vi "getShiftNdDate.vi"(8 "Error In":errorcluster) -> (0 "Error Out":errorcluster, 2 "Production Date":string, 3 "Shift":string)   [LabVIEW 2018]
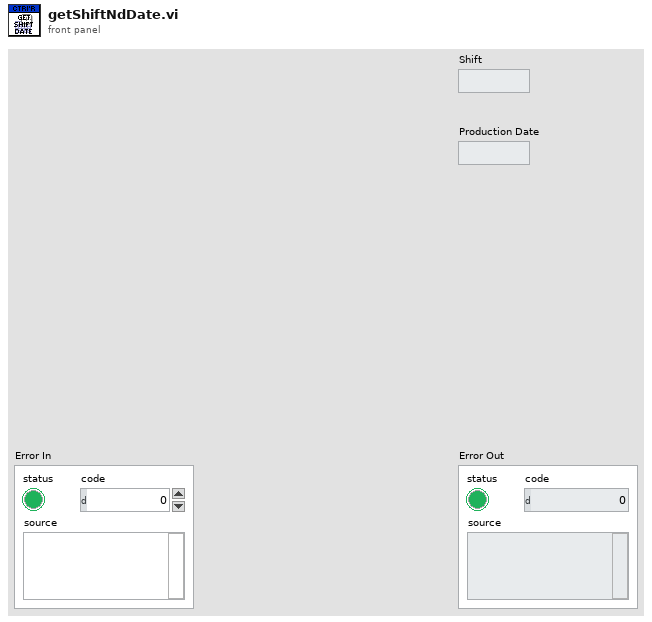
[diagram p1: front panel]
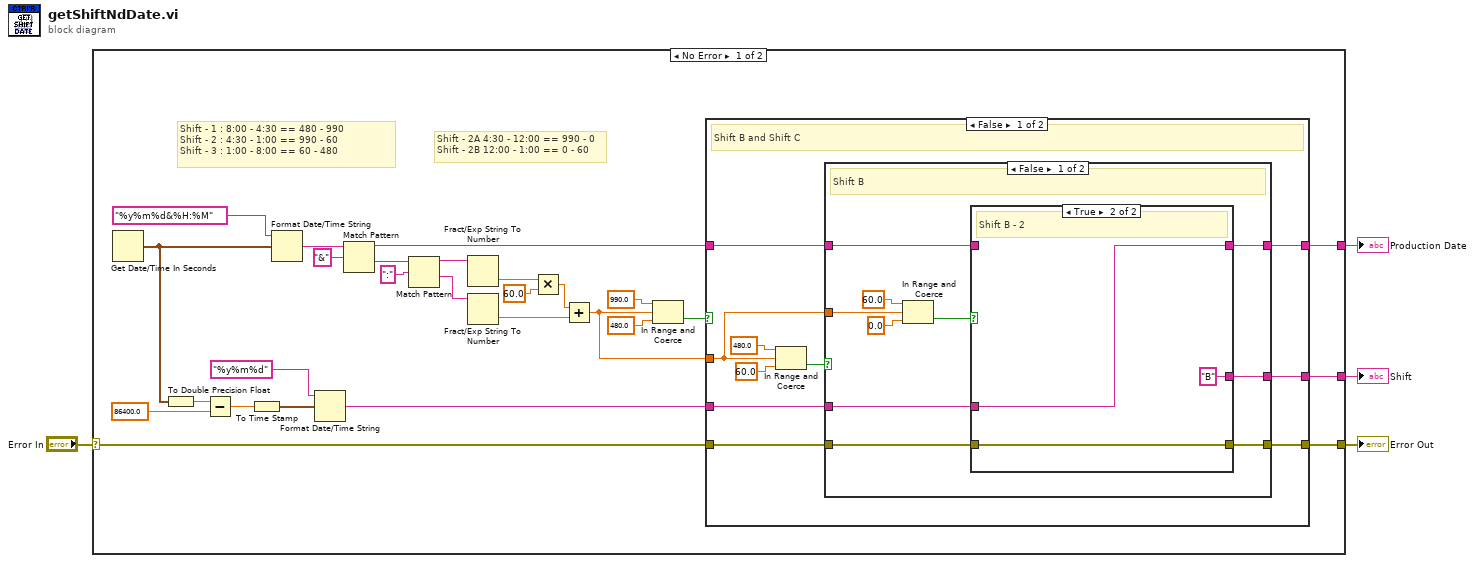
[diagram p0: block diagram]
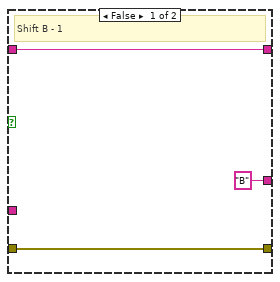
[diagram p2: hidden frame]
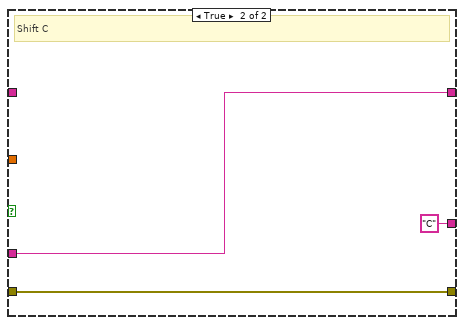
[diagram p3: hidden frame]
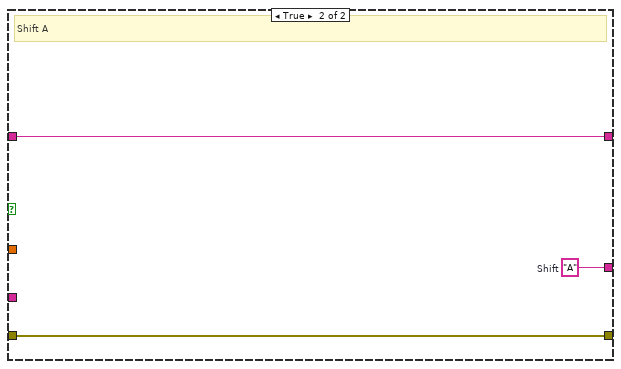
[diagram p4: hidden frame]
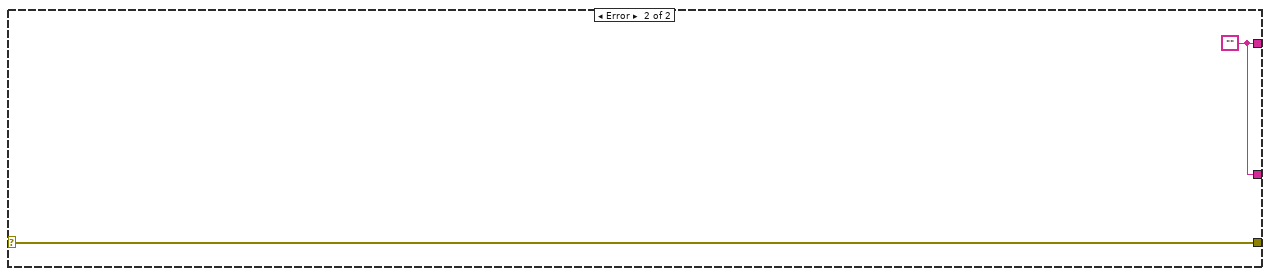
[diagram p5: hidden frame]
diagram:
  n1 = case shown="No Error" "Error In" {
    selector: "Error In" -> [w9 w65]
    tunnel: [w8 w65] -> w3
    tunnel: [w7 w64] -> w2
    tunnel: [w6 w64] -> w1
    frame No Error {
      # "Shift - 2A 4:30 - 12:00 == 990 - 0\nShift - 2B 12:00 - 1:00 == 0 - 60"
      # "Shift - 1 : 8:00 - 4:30 == 480 - 990 \nShift - 2 : 4:30 - 1:00 == 990 - 60 \nShift - 3 : 1:00 - 8:00 == 60 - 480"
      n2 = Get Date/Time In Seconds() -> (seconds since 1Jan1904=w5:timestamp)
      n3 = To Double Precision Float(number=w5) -> (double precision float=w14:dbl)
      n4 = Subtract(x=w14, y=86400.0) -> (x-y=w15:dbl)
      n5 = To Time Stamp(1:w15) -> (0:w12:timestamp)
      n6 = Format Date/Time String(time format string (%c)="%y%m%d&%H:%M", seconds (now)=w5) -> (date/time string=w29:string)  [unwired: 1 in]
      n7 = Format Date/Time String(time format string (%c)="%y%m%d", seconds (now)=w12) -> (date/time string=w10:string)  [unwired: 1 in]
      n8 = Match Pattern(string=w29, regular expression="&" ("search string")) -> (before substring=w16:string, after substring=w21:string)  [unwired: 1 in, 2 out]
      n9 = Match Pattern(string=w21, regular expression=":" ("search string")) -> (before substring=w27:string, after substring=w26:string)  [unwired: 1 in, 2 out]
      n10 = Fract/Exp String To Number(string=w27) -> (number=w25:dbl)  [unwired: 3 in, 1 out]
      n11 = Fract/Exp String To Number(string=w26) -> (number=w22:dbl)  [unwired: 3 in, 1 out]
      n12 = Multiply(x=w25, y=60.0) -> (x*y=w23:dbl)
      n13 = Add(x=w23, y=w22) -> (x+y=w17:dbl)
      n14 = In Range and Coerce(upper limit=990.0, x=w17, lower limit=480.0) -> (In Range?=w18:bool)  [unwired: 1 out]
      n15 = case shown="False" w18 {
        tunnel: w17 -> [w34 _]
        tunnel: w9 -> [w38 w63]
        tunnel: [w39 w63] -> w8
        tunnel: w16 -> [w36 w62]
        tunnel: [w35 w62] -> w6
        tunnel: [w32 w61] -> w7
        tunnel: w10 -> [w33 _]
        frame False {
          # "Shift B and Shift C"
          n16 = In Range and Coerce(upper limit=480.0, x=w34, lower limit=60.0) -> (In Range?=w37:bool)  [unwired: 1 out]
          n17 = case shown="False" w37 {
            tunnel: [w45 w60] -> w39
            tunnel: w38 -> [w44 w60]
            tunnel: w36 -> [w47 _]
            tunnel: [w46 w59] -> w35
            tunnel: w34 -> [w49 _]
            tunnel: w33 -> [w43 w59]
            tunnel: [w42 "C"] -> w32
            frame False {
              # "Shift B"
              n18 = In Range and Coerce(upper limit=60.0, x=w49, lower limit=0.0) -> (In Range?=w48:bool)  [unwired: 1 out]
              n19 = case shown="True" w48 {
                tunnel: w47 -> [w54 _]
                tunnel: [w54 w56] -> w46
                tunnel: [w52 w57] -> w45
                tunnel: w44 -> [w52 w57]
                tunnel: w43 -> [_ w56]
                tunnel: ["B" "B"] -> w42
                frame False {
                  # "Shift B - 1"
                }
                frame True {
                  # "Shift B - 2"
                }
              }
            }
            frame True {
              # "Shift C"
            }
          }
        }
        frame True {
          w61 = "A"  # Shift
          # "Shift A"
        }
      }
    }
    frame Error {
      w64 = ""
    }
  }
  "Error Out" <- w3
  "Shift" <- w2
  "Production Date" <- w1
